vi "HCalGet.vi"(1 "RH?":bool, 2 "Array":u8[][](array[numeric])) -> (0 "Calibration Array":u8[][](array[numeric]))   [LabVIEW 2009]
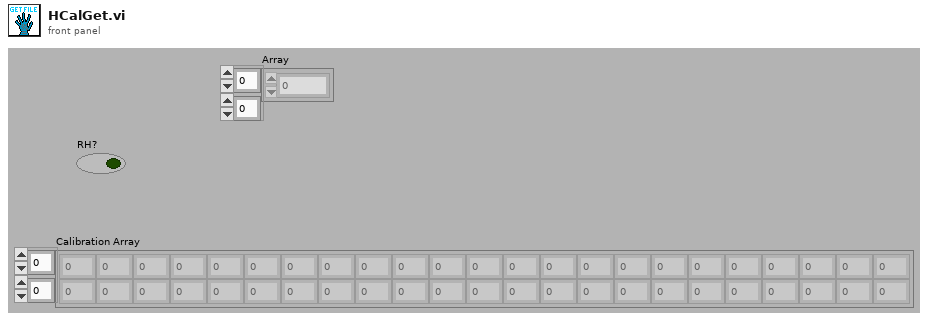
[diagram p1: front panel]
types:
  T1 = enum16{"open", "replace", "create", "open or create", "replace or create", "replace or create with confirmation"}
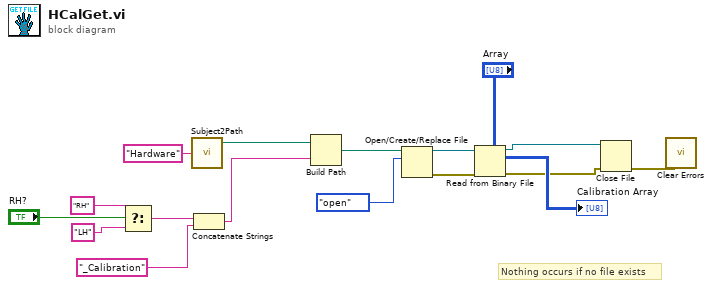
[diagram p0: block diagram]
diagram:
  # "Nothing occurs if no file exists"
  n1 = Select(t="RH" ("name or relative path"), s="RH?", f="LH" ("name or relative path")) -> (s? t:f=w9:string)
  n2 = call "Subject2Path.vi"("Subject Initials"="Hardware") -> ("Subject Root"=w16:path)  [unwired: 1 in, 2 out]
  n3 = Concatenate Strings(w9, "_Calibration" ("name or relative path")) -> (w7:string)
  n4 = Build Path(base path=w16, name or relative path=w7) -> (appended path=w15:path)
  n5 = Open/Create/Replace File(file path (use dialog)=w15, operation (0:open)=T1."open") -> (refnum out=w13:refnum<file>, error out=w3:errorcluster)  [unwired: 4 in, 1 out]
  n6 = Read from Binary File(5:"Array", 8:w3, 11:w13) -> (0:w2:errorcluster, 2:→"Calibration Array":u8[][], 3:w5:refnum<file>)  [unwired: 3 in, 1 out]
  n7 = Close File(refnum=w5, error in=w2) -> (error out=w1:errorcluster)  [unwired: 1 out]
  n8 = call <vilib>:"Clear Errors.vi"("error in (no error)"=w1) -> ()  [unwired: 6 in, 1 out]
